vi "Linear Interpolation GPMtouA.vi"(5 "2D Flow Data (GPM,uA)":dbl[][](array[numeric])=[[0.760276, 4000.0], [0.729117, 4100.0], [0.722886, 4200.0], [0.729117, 4300.0], [0.735349, 4400.0], [0.735349, 4500.0], [0.735349, 4600.0], [0.835058, 4700.0], [0.841289, 4800.0], [0.928534, 4900.0], [0.947229, 5000.0], [1.015779, 5100.0], [1.065633, 5200.0], [1.140414, 5300.0], [1.333599, 5400.0], [1.302441, 5500.0], [1.452003, 5600.0], [1.470698, 5700.0], [1.614029, 5800.0], [1.719969, 5900.0], [1.813446, 6000.0], [2.025326, 6100.0], [2.044021, 6200.0], [2.255902, 6300.0], [2.330683, 6400.0], [2.467782, 6500.0], [2.710821, 6600.0], [2.748212, 6700.0], [2.978787, 6800.0], [2.972556, 6900.0], [3.165741, 7000.0], [3.240522, 7100.0], [3.402548, 7200.0], [3.396316, 7300.0], [3.502256, 7400.0], [3.714137, 7500.0], [3.670514, 7600.0], [3.863699, 7700.0], [3.845004, 7800.0], [4.013262, 7900.0], [4.038189, 8000.0], [4.137897, 8100.0], [4.262533, 8200.0], [4.243837, 8300.0], [4.312387, 8400.0], [4.312387, 8500.0], [4.3934, 8600.0], [4.443254, 8700.0], [4.418327, 8800.0], [4.505572, 8900.0], [4.518035, 9000.0], [4.586585, 9100.0], [4.586585, 9200.0], [4.667598, 9300.0], [4.723684, 9400.0], [4.748611, 9500.0], [4.798465, 9600.0], [4.804697, 9700.0], [4.860783, 9800.0], [4.848319, 9900.0], [4.910637, 10000.0], [4.910637, 10100.0], [4.910637, 10200.0], [4.935564, 10300.0], [4.954259, 10400.0], [5.004114, 10500.0], [5.004114, 10600.0], [4.972955, 10700.0], [5.016577, 10800.0], [5.0602, 10900.0], [5.116285, 11000.0], [5.103822, 11100.0], [5.110054, 11200.0], [5.141213, 11300.0], [5.172371, 11400.0], [5.184835, 11500.0], [5.197299, 11600.0], [5.209762, 11700.0], [5.20353, 11800.0], [5.234689, 11900.0], [5.228457, 12000.0], [5.209762, 12100.0], [5.16614, 12200.0], [5.178603, 12300.0], [5.290775, 12400.0], [5.290775, 12500.0], [5.247153, 12600.0], [5.240921, 12700.0], [5.265848, 12800.0], [5.253384, 12900.0], [5.240921, 13000.0], [5.27208, 13100.0], [5.321934, 13200.0], [5.303239, 13300.0], [5.321934, 13400.0], [5.321934, 13500.0], [5.315702, 13600.0], [5.321934, 13700.0], [5.30947, 13800.0], [5.303239, 13900.0], [5.346861, 14000.0], [5.321934, 14100.0], [5.290775, 14200.0], [5.334398, 14300.0], [5.353093, 14400.0], [5.265848, 14500.0], [5.265848, 14600.0], [5.396715, 14700.0], [5.346861, 14800.0], [5.390483, 14900.0], [5.290775, 15000.0], [5.396715, 15100.0], [5.27208, 15200.0], [5.066431, 15300.0], [5.664682, 15400.0], [5.402947, 15500.0], [5.471497, 15600.0], [5.278312, 15700.0], [5.303239, 15800.0], [5.384252, 15900.0], [5.340629, 16000.0], [5.359325, 16100.0], [5.427874, 16200.0], [5.390483, 16300.0], [5.284543, 16400.0], [5.415411, 16500.0], [5.184835, 16600.0], [5.558741, 16700.0], [4.804697, 16800.0], [5.452801, 16900.0], [5.627291, 17000.0], [5.602364, 17100.0], [5.459033, 17200.0], [5.346861, 17300.0], [5.359325, 17400.0], [5.384252, 17500.0], [5.446569, 17600.0], [5.465265, 17700.0], [5.508887, 17800.0], [5.427874, 17900.0], [5.321934, 18000.0], [5.402947, 18100.0], [5.409179, 18200.0], [5.402947, 18300.0], [5.421642, 18400.0], [5.446569, 18500.0], [5.353093, 18600.0], [5.421642, 18700.0], [5.577437, 18800.0], [5.558741, 18900.0], [5.384252, 19000.0], [5.346861, 19100.0], [5.434106, 19200.0], [5.521351, 19300.0], [5.452801, 19400.0], [5.321934, 19500.0], [5.471497, 19600.0], [5.527583, 19700.0], [5.353093, 19800.0], [5.353093, 19900.0], [5.396715, 20000.0]], 10 "GPM Target":dbl) -> (2 "uA Output":i32)   [LabVIEW 2012]
uses:
  <vilib>/gmath/NI_Gmath.lvlib
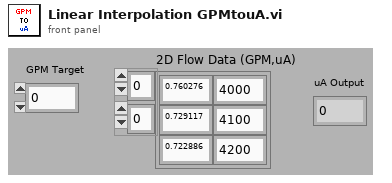
[diagram p1: front panel]
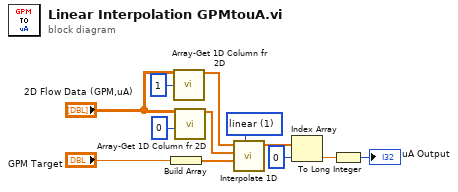
[diagram p0: block diagram]
diagram:
  w11 = 1 items=["nearest", "linear", "spline", "cubic Hermite", "Lagrange"] ("method")
  n1 = Build Array("GPM Target") -> (w8:dbl[])
  n2 = call "Array-Get 1D Column fr 2D.vi"("2D Array Data"="2D Flow Data (GPM,uA)", "column index"=1) -> ("Column Data"=w1:dbl[])  [unwired: 13 in]
  n3 = call "Array-Get 1D Column fr 2D.vi"("2D Array Data"="2D Flow Data (GPM,uA)", "column index"=0) -> ("Column Data"=w2:dbl[])  [unwired: 13 in]
  n4 = call <vilib>:"Interpolate 1D.vi"("method"=w11, "xi"=w8, "X"=w2, "Y"=w1) -> ("yi"=w7:dbl[])  [unwired: 5 in, 2 out]
  n5 = Index Array(array=w7, index=0) -> (element=w3:dbl)
  n6 = To Long Integer(number=w3) -> (32bit integer=→"uA Output":i32)
